vi "myRIO_BRig_RT__Case_Exp_State_initTrial_LC_ENL1__v4.vi"(6 "input_dataTrial":u16[][](array[numeric]), 7 "input_spout":enum16{"Left", "Right"}(ring), 8 "input_arrTrig":bool[](array[boolean]), 9 "input_dataBlock":u16[][](array[numeric]), 10 "input_dataLC":u16[](array[numeric]), 11 "input_dataCurrent":u16[](array[numeric])) -> (0 "output_arrTrig":bool[](array[boolean]), 4 "output_dataTrial":u16[][](array[numeric]), 5 "output_dataCurrent":u16[](array[numeric]))   [LabVIEW 2014]
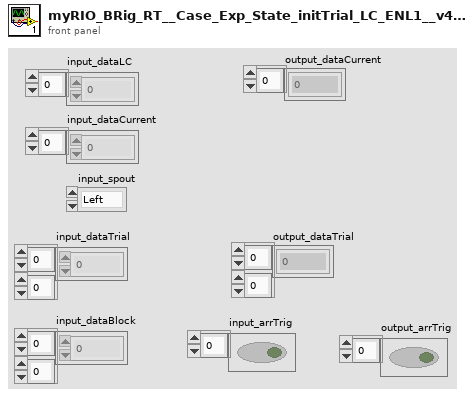
[diagram p1: front panel]
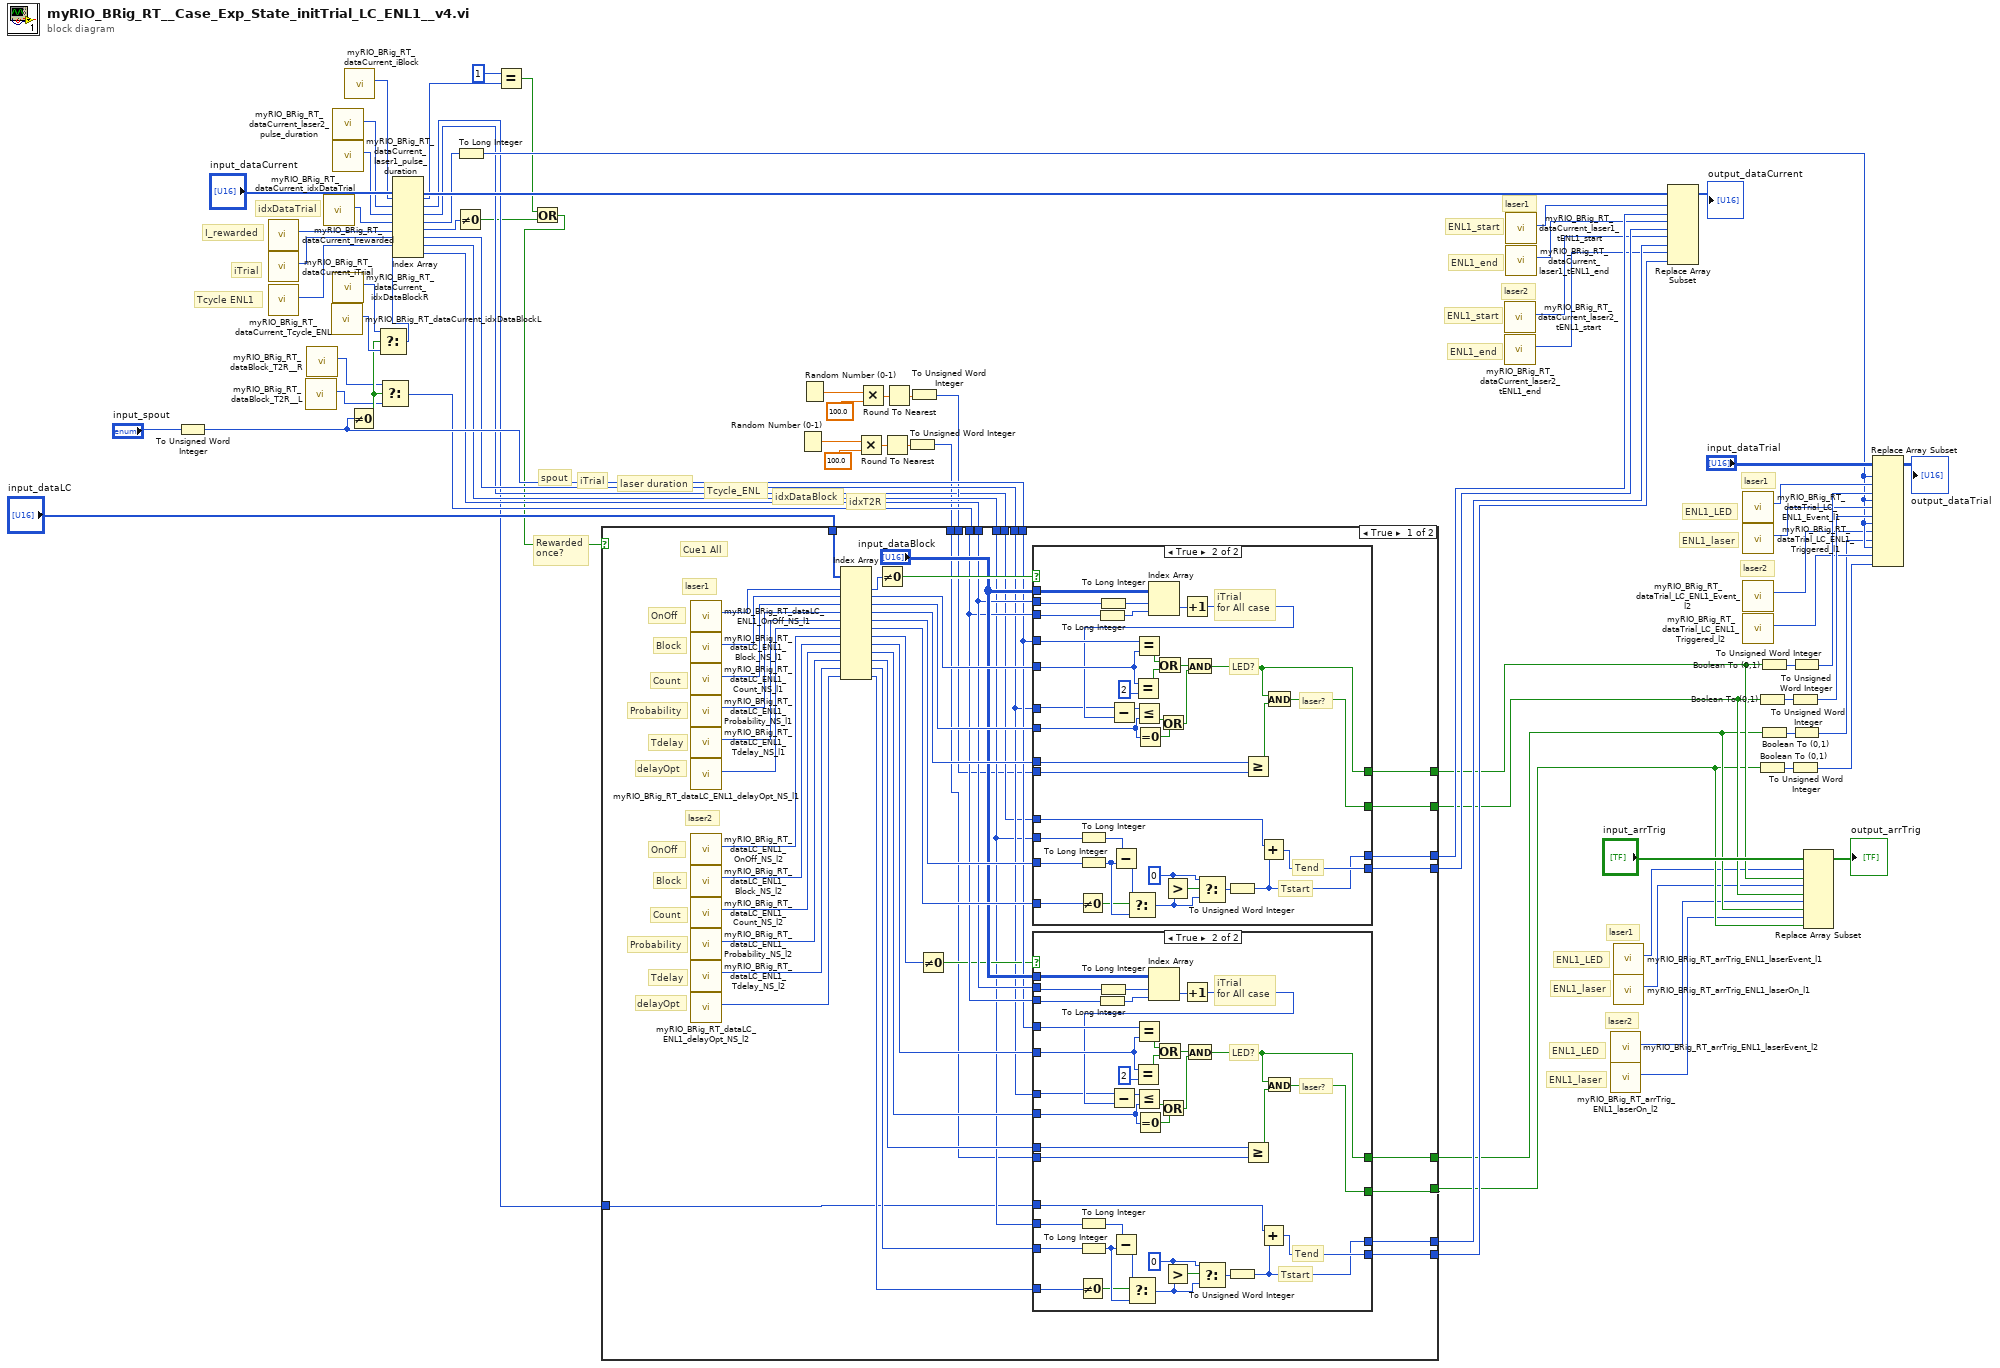
[diagram p0: block diagram]
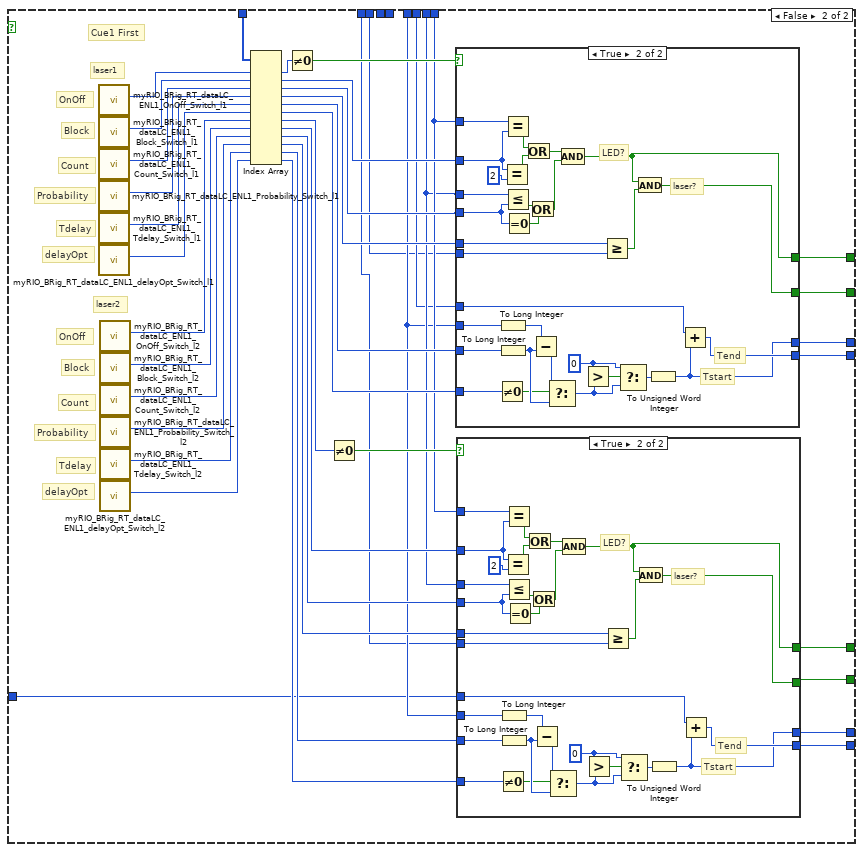
[diagram p4: hidden frame]
diagram:
  # "ENL1_LED"
  # "ENL1_laser"
  # "ENL1_end"
  # "ENL1_start"
  # "ENL1_end"
  # "ENL1_start"
  # "ENL1_LED"
  # "ENL1_laser"
  # "ENL1_LED"
  # "ENL1_laser"
  # "laser2"
  # "laser1"
  # "laser2"
  # "laser1"
  # "laser2"
  # "laser1"
  # "idxT2R"
  # "idxDataBlock"
  # "Tcycle_ENL"
  # "laser duration"
  # "iTrial"
  # "spout"
  # "Rewarded\nonce?"
  # "iTrial"
  # "idxDataTrial"
  # "Tcycle ENL1"
  # "I_rewarded"
  n1 = To Unsigned Word Integer(number="input_spout") -> (unsigned 16bit integer=w51:u16)
  n2 = call "myRIO_BRig_RT_dataCurrent_Irewarded.vi"() -> ("output_I_rewarded"=w72:i32)  [unwired: 11 in]
  n3 = call "myRIO_BRig_RT_dataCurrent_iTrial.vi"() -> ("output_iTrial"=w61:i32)  [unwired: 11 in]
  n4 = call "myRIO_BRig_RT_dataCurrent_Tcycle_ENL.vi"() -> ("output_ENL"=w31:i32)  [unwired: 11 in]
  n5 = call "myRIO_BRig_RT_dataBlock_T2R__L.vi"() -> ("output_T2R__L"=w55:i32)  [unwired: 11 in]
  n6 = call "myRIO_BRig_RT_dataBlock_T2R__R.vi"() -> ("output_T2R__R"=w56:i32)  [unwired: 11 in]
  n7 = call "myRIO_BRig_RT_dataCurrent_idxDataTrial.vi"() -> ("output_idxDataTrial"=w65:i32)  [unwired: 11 in]
  n8 = call "myRIO_BRig_RT_dataCurrent_idxDataBlockL.vi"() -> ("output_idxDataBlock__L"=w60:i32)  [unwired: 11 in]
  n9 = call "myRIO_BRig_RT_dataCurrent_laser2_pulse_duration.vi"() -> ("output_laser2_pulse_duration"=w15:i32)  [unwired: 11 in]
  n10 = call "myRIO_BRig_RT_dataCurrent_laser1_pulse_duration.vi"() -> ("output_laser1_pulse_duration"=w14:i32)  [unwired: 11 in]
  n11 = call "myRIO_BRig_RT_dataCurrent_idxDataBlockR.vi"() -> ("output_idxDataBlock__R"=w59:i32)  [unwired: 11 in]
  n12 = call "myRIO_BRig_RT_dataCurrent_iBlock.vi"() -> ("output_iBlock"=w6:i32)  [unwired: 11 in]
  n13 = Not Equal To 0?(x=w51) -> (x != 0?=w57:bool)
  n14 = Select(t=w59, s=w57, f=w60) -> (s? t:f=w58:i32)
  n15 = Select(t=w56, s=w57, f=w55) -> (s? t:f=w47:i32)
  n16 = Index Array(array="input_dataCurrent", index #1=w6, index #2=w15, index #3=w14, index #4=w65, index #5=w72, index #6=w61, index #7=w31, index #8=w58) -> (element #1=w5:u16, element #2=w12:u16, element #3=w13:u16, element #4=w64:u16, element #5=w73:u16, element #6=w50:u16, element #7=w49:u16, element #8=w48:u16)
  n17 = Not Equal To 0?(x=w73) -> (x != 0?=w3:bool)
  n18 = To Long Integer(number=w64) -> (32bit integer=w20:i32)
  n19 = Equal?(x=u16 1, y=w5) -> (x = y?=w2:bool)
  n20 = Or(x=w2, y=w3) -> (x .or. y?=w1:bool)
  n21 = Random Number (0-1)() -> (number: 0 to 1=w8:dbl)
  n22 = Random Number (0-1)() -> (number: 0 to 1=w43:dbl)
  n23 = Multiply(x=w8, y=100.0) -> (x*y=w9:dbl)
  n24 = Multiply(x=w43, y=100.0) -> (x*y=w44:dbl)
  n25 = Round To Nearest(number=w9) -> (nearest integer value=w10:dbl)
  n26 = Round To Nearest(number=w44) -> (nearest integer value=w45:dbl)
  n27 = To Unsigned Word Integer(number=w10) -> (unsigned 16bit integer=w7:u16)
  n28 = To Unsigned Word Integer(number=w45) -> (unsigned 16bit integer=w42:u16)
  n29 = case shown="True" w1 {
    tunnel: "input_dataLC" -> [w119 w237]
    tunnel: w51 -> [w108 w219]
    tunnel: w50 -> [w104 w217]
    tunnel: w13 -> [w101 w214]
    tunnel: w49 -> [w100 w213]
    tunnel: w48 -> [w110 _]
    tunnel: w47 -> [w109 _]
    tunnel: w42 -> [w75 w196]
    tunnel: [w97 w228] -> w35
    tunnel: [w96 w227] -> w34
    tunnel: [w95 w226] -> w41
    tunnel: [w94 w225] -> w40
    tunnel: [w93 w223] -> w33
    tunnel: [w92 w222] -> w32
    tunnel: [w91 w221] -> w39
    tunnel: [w90 w220] -> w38
    tunnel: w12 -> [w89 w210]
    tunnel: w7 -> [w76 w197]
    frame True {
      # "laser2"
      # "laser1"
      # "delayOpt"
      # "Count"
      # "Tdelay"
      # "Probability"
      # "OnOff"
      # "Block"
      # "delayOpt"
      # "Count"
      # "Tdelay"
      # "Probability"
      # "OnOff"
      # "Block"
      # "Cue1 All"
      n30 = call "myRIO_BRig_RT_dataLC_ENL1_OnOff_NS_l1.vi"() -> ("output_ENL1_OnOff_NS_l1"=w88:i32)  [unwired: 11 in]
      n31 = call "myRIO_BRig_RT_dataLC_ENL1_Block_NS_l1.vi"() -> ("output_ENL1_All_Block"=w87:i32)  [unwired: 11 in]
      n32 = call "myRIO_BRig_RT_dataLC_ENL1_Count_NS_l1.vi"() -> ("output_ENL1_Count_NS_l1"=w86:i32)  [unwired: 11 in]
      n33 = call "myRIO_BRig_RT_dataLC_ENL1_Probability_NS_l1.vi"() -> ("output_ENL1_Probability_NS_l1"=w85:i32)  [unwired: 11 in]
      n34 = call "myRIO_BRig_RT_dataLC_ENL1_Tdelay_NS_l1.vi"() -> ("output_ENL1_Tdelay_NS_l1"=w84:i32)  [unwired: 11 in]
      n35 = call "myRIO_BRig_RT_dataLC_ENL1_delayOpt_NS_l1.vi"() -> ("output_ENL1_delayOpt_NS_l1"=w83:i32)  [unwired: 11 in]
      n36 = call "myRIO_BRig_RT_dataLC_ENL1_OnOff_NS_l2.vi"() -> ("output_ENL1_OnOff_NS_l2"=w82:i32)  [unwired: 11 in]
      n37 = call "myRIO_BRig_RT_dataLC_ENL1_Block_NS_l2.vi"() -> ("output_ENL1_Block_NS_l2"=w81:i32)  [unwired: 11 in]
      n38 = call "myRIO_BRig_RT_dataLC_ENL1_Count_NS_l2.vi"() -> ("output_ENL1_Count_NS_l2"=w80:i32)  [unwired: 11 in]
      n39 = call "myRIO_BRig_RT_dataLC_ENL1_Probability_NS_l2.vi"() -> ("output_ENL1_Probability_NS_l2"=w79:i32)  [unwired: 11 in]
      n40 = call "myRIO_BRig_RT_dataLC_ENL1_Tdelay_NS_l2.vi"() -> ("output_ENL1_Tdelay_NS_l2"=w78:i32)  [unwired: 11 in]
      n41 = call "myRIO_BRig_RT_dataLC_ENL1_delayOpt_NS_l2.vi"() -> ("output_ENL1_delayOpt_NS_l2"=w77:i32)  [unwired: 11 in]
      n42 = Index Array(array=w119, index #1=w88, index #2=w87, index #3=w86, index #4=w85, index #5=w84, index #6=w83, index #7=w82, index #8=w81, index #9=w80, index #10=w79, index #11=w78, index #12=w77) -> (element #1=w114:u16, element #2=w112:u16, element #3=w118:u16, element #4=w117:u16, element #5=w116:u16, element #6=w115:u16, element #7=w107:u16, element #8=w105:u16, element #9=w103:u16, element #10=w102:u16, element #11=w99:u16, element #12=w98:u16)
      n43 = Not Equal To 0?(x=w114) -> (x != 0?=w113:bool)
      n44 = Not Equal To 0?(x=w107) -> (x != 0?=w106:bool)
      n45 = case shown="True" w113 {
        tunnel: w108 -> [_ w194]
        tunnel: w104 -> [_ w179]
        tunnel: [_ w174] -> w97
        tunnel: [_ w190] -> w96
        tunnel: [_ w165] -> w94
        tunnel: [_ w164] -> w95
        tunnel: w101 -> [_ w163]
        tunnel: w100 -> [_ w162]
        tunnel: w109 -> [_ w185]
        tunnel: w110 -> [_ w187]
        tunnel: w112 -> [_ w182]
        tunnel: w118 -> [_ w181]
        tunnel: w117 -> [_ w177]
        tunnel: w116 -> [_ w161]
        tunnel: w115 -> [_ w160]
        tunnel: "input_dataBlock" -> [_ w159]
        tunnel: w75 -> [_ w158]
        frame False {
        }
        frame True {
          w171 = 0 ("x")
          # "Tstart"
          # "Tend"
          # "iTrial\nfor All case"
          # "laser?"
          # "LED?"
          n46 = Not Equal To 0?(x=w160) -> (x != 0?=w168:bool)
          n47 = To Long Integer(number=w162) -> (32bit integer=w166:i32)
          n48 = To Long Integer(number=w161) -> (32bit integer=w169:i32)
          n49 = To Long Integer(number=w185) -> (32bit integer=w184:i32)
          n50 = To Long Integer(number=w187) -> (32bit integer=w186:i32)
          n51 = Subtract(x=w166, y=w169) -> (x-y=w167:i32)
          n52 = Select(t=w167, s=w168, f=w169) -> (s? t:f=w172:i32)
          n53 = Equal?(x=w182, y=u16 2) -> (x = y?=w192:bool)
          n54 = Equal?(x=w194, y=w182) -> (x = y?=w193:bool)
          n55 = Equal To 0?(x=w181) -> (x = 0?=w188:bool)
          n56 = Index Array(array=w159, index (row)=w186, index (col)=w184) -> (element=w183:u16)
          n57 = Or(x=w193, y=w192) -> (x .or. y?=w176:bool)
          n58 = Greater?(x=w171, y=w172) -> (0:w170:bool)
          n59 = Increment(x=w183) -> (x+1=w180:u16)
          n60 = Subtract(x=w179, y=w180) -> (x-y=w178:u16)
          n61 = Less Or Equal?(x=w178, y=w181) -> (x <= y?=w189:bool)
          n62 = Or(x=w189, y=w188) -> (x .or. y?=w175:bool)
          n63 = And(x=w176, y=w175) -> (x .and. y?=w174:bool)
          n64 = Select(t=w171, s=w170, f=w172) -> (s? t:f=w173:i32)
          n65 = To Unsigned Word Integer(number=w173) -> (unsigned 16bit integer=w164:u16)
          n66 = Greater Or Equal?(x=w177, y=w158) -> (x >= y?=w191:bool)
          n67 = Add(x=w163, y=w164) -> (x+y=w165:u16)
          n68 = And(x=w174, y=w191) -> (x .and. y?=w190:bool)
        }
      }
      n69 = case shown="True" w106 {
        tunnel: w108 -> [_ w156]
        tunnel: w104 -> [_ w141]
        tunnel: [_ w136] -> w93
        tunnel: [_ w152] -> w92
        tunnel: [_ w127] -> w90
        tunnel: [_ w126] -> w91
        tunnel: w89 -> [_ w125]
        tunnel: w100 -> [_ w124]
        tunnel: w109 -> [_ w147]
        tunnel: w110 -> [_ w149]
        tunnel: w105 -> [_ w144]
        tunnel: w103 -> [_ w143]
        tunnel: w102 -> [_ w139]
        tunnel: w99 -> [_ w123]
        tunnel: w98 -> [_ w122]
        tunnel: "input_dataBlock" -> [_ w121]
        tunnel: w76 -> [_ w120]
        frame False {
        }
        frame True {
          w133 = 0 ("x")
          # "Tstart"
          # "Tend"
          # "iTrial\nfor All case"
          # "laser?"
          # "LED?"
          n70 = Not Equal To 0?(x=w122) -> (x != 0?=w130:bool)
          n71 = To Long Integer(number=w124) -> (32bit integer=w128:i32)
          n72 = To Long Integer(number=w123) -> (32bit integer=w131:i32)
          n73 = To Long Integer(number=w147) -> (32bit integer=w146:i32)
          n74 = To Long Integer(number=w149) -> (32bit integer=w148:i32)
          n75 = Subtract(x=w128, y=w131) -> (x-y=w129:i32)
          n76 = Select(t=w129, s=w130, f=w131) -> (s? t:f=w134:i32)
          n77 = Equal?(x=w144, y=u16 2) -> (x = y?=w154:bool)
          n78 = Equal?(x=w156, y=w144) -> (x = y?=w155:bool)
          n79 = Equal To 0?(x=w143) -> (x = 0?=w150:bool)
          n80 = Index Array(array=w121, index (row)=w148, index (col)=w146) -> (element=w145:u16)
          n81 = Or(x=w155, y=w154) -> (x .or. y?=w138:bool)
          n82 = Greater?(x=w133, y=w134) -> (0:w132:bool)
          n83 = Increment(x=w145) -> (x+1=w142:u16)
          n84 = Subtract(x=w141, y=w142) -> (x-y=w140:u16)
          n85 = Less Or Equal?(x=w140, y=w143) -> (x <= y?=w151:bool)
          n86 = Or(x=w151, y=w150) -> (x .or. y?=w137:bool)
          n87 = And(x=w138, y=w137) -> (x .and. y?=w136:bool)
          n88 = Select(t=w133, s=w132, f=w134) -> (s? t:f=w135:i32)
          n89 = To Unsigned Word Integer(number=w135) -> (unsigned 16bit integer=w126:u16)
          n90 = Greater Or Equal?(x=w139, y=w120) -> (x >= y?=w153:bool)
          n91 = Add(x=w125, y=w126) -> (x+y=w127:u16)
          n92 = And(x=w136, y=w153) -> (x .and. y?=w152:bool)
        }
      }
    }
    frame False {
      # "laser2"
      # "laser1"
      # "delayOpt"
      # "Count"
      # "Tdelay"
      # "Probability"
      # "OnOff"
      # "Block"
      # "delayOpt"
      # "Count"
      # "Tdelay"
      # "Probability"
      # "OnOff"
      # "Block"
      # "Cue1 First"
      n93 = call "myRIO_BRig_RT_dataLC_ENL1_OnOff_Switch_l1.vi"() -> ("output_ENL1_OnOff_Switch_l1"=w209:i32)  [unwired: 11 in]
      n94 = call "myRIO_BRig_RT_dataLC_ENL1_Block_Switch_l1.vi"() -> ("output_ENL1_Block_Switch_l1"=w208:i32)  [unwired: 11 in]
      n95 = call "myRIO_BRig_RT_dataLC_ENL1_Count_Switch_l1.vi"() -> ("output_ENL1_Count_Switch_l1"=w207:i32)  [unwired: 11 in]
      n96 = call "myRIO_BRig_RT_dataLC_ENL1_Probability_Switch_l1.vi"() -> ("output_ENL1_Probability_Switch_l1"=w206:i32)  [unwired: 11 in]
      n97 = call "myRIO_BRig_RT_dataLC_ENL1_Tdelay_Switch_l1.vi"() -> ("output_ENL1_Tdelay_Switch_l1"=w205:i32)  [unwired: 11 in]
      n98 = call "myRIO_BRig_RT_dataLC_ENL1_delayOpt_Switch_l1.vi"() -> ("output_ENL1_delayOpt_Switch_l1"=w204:i32)  [unwired: 11 in]
      n99 = call "myRIO_BRig_RT_dataLC_ENL1_OnOff_Switch_l2.vi"() -> ("output_ENL1_OnOff_Switch_l2"=w203:i32)  [unwired: 11 in]
      n100 = call "myRIO_BRig_RT_dataLC_ENL1_Block_Switch_l2.vi"() -> ("output_ENL1_Block_Switch_l2"=w202:i32)  [unwired: 11 in]
      n101 = call "myRIO_BRig_RT_dataLC_ENL1_Count_Switch_l2.vi"() -> ("output_ENL1_Count_Switch_l2"=w201:i32)  [unwired: 11 in]
      n102 = call "myRIO_BRig_RT_dataLC_ENL1_Probability_Switch_l2.vi"() -> ("output_ENL1_Probability_Switch_l2"=w200:i32)  [unwired: 11 in]
      n103 = call "myRIO_BRig_RT_dataLC_ENL1_Tdelay_Switch_l2.vi"() -> ("output_ENL1_Tdelay_Switch_l2"=w199:i32)  [unwired: 11 in]
      n104 = call "myRIO_BRig_RT_dataLC_ENL1_delayOpt_Switch_l2.vi"() -> ("output_ENL1_delayOpt_Switch_l2"=w198:i32)  [unwired: 11 in]
      n105 = Index Array(array=w237, index #1=w209, index #2=w208, index #3=w207, index #4=w206, index #5=w205, index #6=w204, index #7=w203, index #8=w202, index #9=w201, index #10=w200, index #11=w199, index #12=w198) -> (element #1=w236:u16, element #2=w232:u16, element #3=w231:u16, element #4=w233:u16, element #5=w230:u16, element #6=w229:u16, element #7=w235:u16, element #8=w218:u16, element #9=w216:u16, element #10=w215:u16, element #11=w212:u16, element #12=w211:u16)
      n106 = Not Equal To 0?(x=w236) -> (x != 0?=w234:bool)
      n107 = Not Equal To 0?(x=w235) -> (x != 0?=w224:bool)
      n108 = case shown="True" w234 {
        tunnel: w219 -> [_ w296]
        tunnel: w232 -> [_ w295]
        tunnel: w217 -> [_ w294]
        tunnel: [_ w289] -> w228
        tunnel: [_ w288] -> w227
        tunnel: [_ w271] -> w225
        tunnel: w229 -> [_ w275]
        tunnel: w230 -> [_ w274]
        tunnel: [_ w270] -> w226
        tunnel: w231 -> [_ w287]
        tunnel: w213 -> [_ w273]
        tunnel: w214 -> [_ w272]
        tunnel: w196 -> [_ w269]
        tunnel: w233 -> [_ w268]
        frame False {
        }
        frame True {
          w281 = 0 ("x")
          # "Tstart"
          # "Tend"
          # "laser?"
          # "LED?"
          n109 = Not Equal To 0?(x=w275) -> (x != 0?=w278:bool)
          n110 = To Long Integer(number=w273) -> (32bit integer=w276:i32)
          n111 = To Long Integer(number=w274) -> (32bit integer=w279:i32)
          n112 = Equal?(x=w295, y=u16 2) -> (x = y?=w292:bool)
          n113 = Equal?(x=w296, y=w295) -> (x = y?=w293:bool)
          n114 = Less Or Equal?(x=w294, y=w287) -> (x <= y?=w286:bool)
          n115 = Equal To 0?(x=w287) -> (x = 0?=w285:bool)
          n116 = Or(x=w293, y=w292) -> (x .or. y?=w291:bool)
          n117 = Or(x=w286, y=w285) -> (x .or. y?=w284:bool)
          n118 = Subtract(x=w276, y=w279) -> (x-y=w277:i32)
          n119 = Select(t=w277, s=w278, f=w279) -> (s? t:f=w282:i32)
          n120 = Compound Arithmetic op=AND(w291, w284) -> (w289:bool)
          n121 = Greater?(x=w281, y=w282) -> (0:w280:bool)
          n122 = Greater Or Equal?(x=w268, y=w269) -> (x >= y?=w290:bool)
          n123 = Select(t=w281, s=w280, f=w282) -> (s? t:f=w283:i32)
          n124 = And(x=w289, y=w290) -> (x .and. y?=w288:bool)
          n125 = To Unsigned Word Integer(number=w283) -> (unsigned 16bit integer=w270:u16)
          n126 = Add(x=w272, y=w270) -> (x+y=w271:u16)
        }
      }
      n127 = case shown="True" w224 {
        tunnel: w219 -> [_ w266]
        tunnel: w218 -> [_ w265]
        tunnel: w217 -> [_ w264]
        tunnel: [_ w259] -> w223
        tunnel: [_ w258] -> w222
        tunnel: [_ w241] -> w220
        tunnel: w211 -> [_ w245]
        tunnel: w212 -> [_ w244]
        tunnel: [_ w240] -> w221
        tunnel: w216 -> [_ w257]
        tunnel: w213 -> [_ w243]
        tunnel: w210 -> [_ w242]
        tunnel: w197 -> [_ w239]
        tunnel: w215 -> [_ w238]
        frame False {
        }
        frame True {
          w251 = 0 ("x")
          # "Tstart"
          # "Tend"
          # "laser?"
          # "LED?"
          n128 = Not Equal To 0?(x=w245) -> (x != 0?=w248:bool)
          n129 = To Long Integer(number=w243) -> (32bit integer=w246:i32)
          n130 = To Long Integer(number=w244) -> (32bit integer=w249:i32)
          n131 = Equal?(x=w265, y=u16 2) -> (x = y?=w262:bool)
          n132 = Equal?(x=w266, y=w265) -> (x = y?=w263:bool)
          n133 = Less Or Equal?(x=w264, y=w257) -> (x <= y?=w256:bool)
          n134 = Equal To 0?(x=w257) -> (x = 0?=w255:bool)
          n135 = Or(x=w263, y=w262) -> (x .or. y?=w261:bool)
          n136 = Or(x=w256, y=w255) -> (x .or. y?=w254:bool)
          n137 = Subtract(x=w246, y=w249) -> (x-y=w247:i32)
          n138 = Select(t=w247, s=w248, f=w249) -> (s? t:f=w252:i32)
          n139 = Compound Arithmetic op=AND(w261, w254) -> (w259:bool)
          n140 = Greater?(x=w251, y=w252) -> (0:w250:bool)
          n141 = Greater Or Equal?(x=w238, y=w239) -> (x >= y?=w260:bool)
          n142 = Select(t=w251, s=w250, f=w252) -> (s? t:f=w253:i32)
          n143 = And(x=w259, y=w260) -> (x .and. y?=w258:bool)
          n144 = To Unsigned Word Integer(number=w253) -> (unsigned 16bit integer=w240:u16)
          n145 = Add(x=w242, y=w240) -> (x+y=w241:u16)
        }
      }
    }
  }
  n146 = call "myRIO_BRig_RT_dataCurrent_laser2_tENL1_start.vi"() -> ("output_laser2_tENL1_start"=w28:i32)  [unwired: 11 in]
  n147 = call "myRIO_BRig_RT_dataCurrent_laser2_tENL1_end.vi"() -> ("output_laser2_tENL1_end"=w27:i32)  [unwired: 11 in]
  n148 = call "myRIO_BRig_RT_dataCurrent_laser1_tENL1_start.vi"() -> ("output_laser1_tENL1_start"=w30:i32)  [unwired: 11 in]
  n149 = call "myRIO_BRig_RT_dataCurrent_laser1_tENL1_end.vi"() -> ("output_laser1_tENL1_end"=w29:i32)  [unwired: 11 in]
  n150 = call "myRIO_BRig_RT_arrTrig_ENL1_laserEvent_l2.vi"() -> ("output_arrTrig_ENL1_laserEvent_l2"=w22:i32)  [unwired: 11 in]
  n151 = call "myRIO_BRig_RT_arrTrig_ENL1_laserOn_l2.vi"() -> ("output_arrTrig_ENL1_laserOn_l2"=w21:i32)  [unwired: 11 in]
  n152 = call "myRIO_BRig_RT_arrTrig_ENL1_laserEvent_l1.vi"() -> ("output_arrTrig_ENL1_laserEvent_l1"=w24:i32)  [unwired: 11 in]
  n153 = call "myRIO_BRig_RT_arrTrig_ENL1_laserOn_l1.vi"() -> ("output_arrTrig_ENL1_laserOn_l1"=w23:i32)  [unwired: 11 in]
  n154 = Replace Array Subset(array="input_dataCurrent", new element #1=w41, index #1=w30, new element #2=w40, index #2=w29, new element #3=w39, index #3=w28, new element #4=w38, index #4=w27) -> (→"output_dataCurrent":u16[])
  n155 = call "myRIO_BRig_RT_dataTrial_LC_ENL1_Event_l1.vi"() -> ("output_LC_ENL1_Event_l1"=w26:i32)  [unwired: 11 in]
  n156 = call "myRIO_BRig_RT_dataTrial_LC_ENL1_Triggered_l1.vi"() -> ("output_LC_ENL1_Triggered_l1"=w25:i32)  [unwired: 11 in]
  n157 = call "myRIO_BRig_RT_dataTrial_LC_ENL1_Event_l2.vi"() -> ("output_LC_ENL1_Event_l2"=w19:i32)  [unwired: 11 in]
  n158 = call "myRIO_BRig_RT_dataTrial_LC_ENL1_Triggered_l2.vi"() -> ("output_LC_ENL1_Triggered_l2"=w18:i32)  [unwired: 11 in]
  n159 = Boolean To (0,1)(Boolean=w34) -> (0, 1=w68:i16)
  n160 = Boolean To (0,1)(Boolean=w32) -> (0, 1=w37:i16)
  n161 = Boolean To (0,1)(Boolean=w35) -> (0, 1=w69:i16)
  n162 = Boolean To (0,1)(Boolean=w33) -> (0, 1=w36:i16)
  n163 = To Unsigned Word Integer(number=w68) -> (unsigned 16bit integer=w62:u16)
  n164 = To Unsigned Word Integer(number=w37) -> (unsigned 16bit integer=w16:u16)
  n165 = To Unsigned Word Integer(number=w69) -> (unsigned 16bit integer=w63:u16)
  n166 = To Unsigned Word Integer(number=w36) -> (unsigned 16bit integer=w17:u16)
  n167 = Replace Array Subset(array="input_arrTrig", new element #1=w35, index #1=w24, new element #2=w34, index #2=w23, new element #3=w33, index #3=w22, new element #4=w32, index #4=w21) -> (→"output_arrTrig":bool[])
  n168 = Replace Array Subset(array="input_dataTrial", new element #1=w63, index (row) #1=w20, index (col) #1=w26, new element #2=w62, index (row) #2=w20, index (col) #2=w25, new element #3=w17, index (row) #3=w20, index (col) #3=w19, new element #4=w16, index (row) #4=w20, index (col) #4=w18) -> (→"output_dataTrial":u16[][])
